vi "Addon.Dialog.vi"(8 "error in (no error)":errorcluster) -> (0 "error out":errorcluster, 2 "Diagnostics Basic Configuration":T1, 3 "Cancelled?":bool)   [LabVIEW 2024, in "Diagnostics Addon System Explorer.lvlib"]
uses:
  Diagnostics Addon System Explorer.lvlib
  Addon Shared/Types/Protocol.ctl
  Types/Addon.Initialize.ctl
  Addon Shared/Diagnostics Addon Shared.lvlib
panel:
  in  "Baud Rate":u32=250000
  in  "Path":path caption="Previous Personality Path (Optional)"
  in  "Cancel":bool
  in  "OK":bool
  in  "Diagnostic Protocol":T2
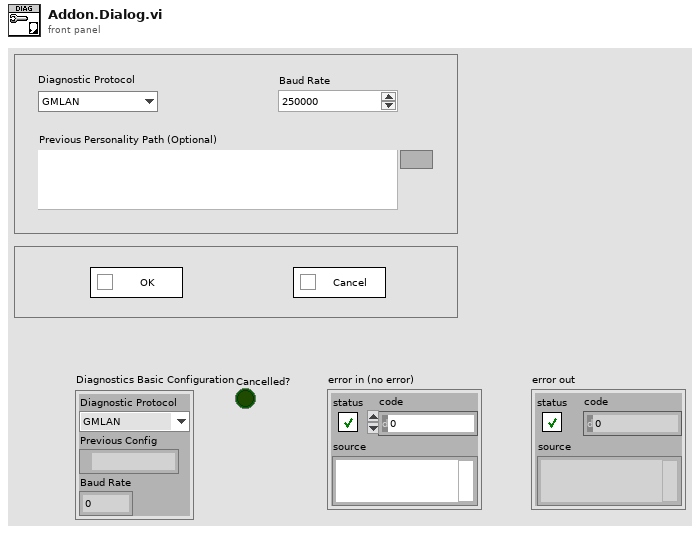
[diagram p1: front panel]
types:
  T1 = typedef "Diagnostics Addon System Explorer.lvlib/Addon.Initialize.ctl" = cluster{"Diagnostic Protocol":T2, "Previous Config":path, "Baud Rate":u32}
  T2 = typedef "Diagnostics Addon Shared.lvlib/Protocol.ctl" = enum16{"GMLAN", "KWP-2000", "UDS", "User-Defined"}
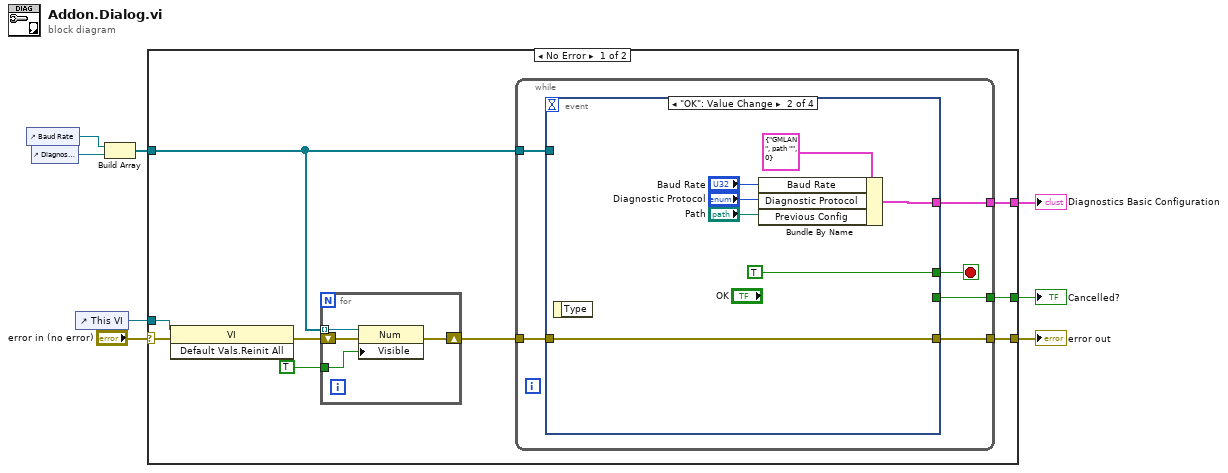
[diagram p0: block diagram]
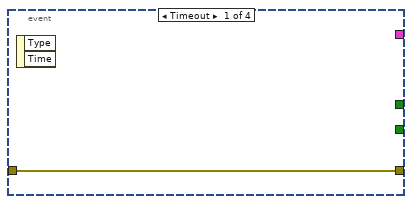
[diagram p2: hidden frame]
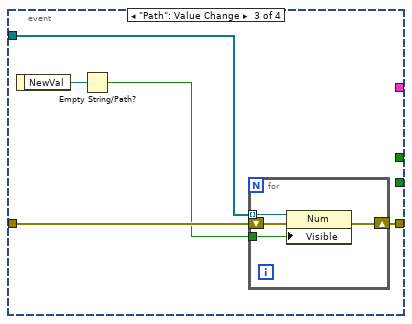
[diagram p3: hidden frame]
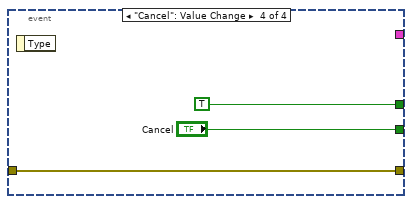
[diagram p4: hidden frame]
diagram:
  n1 = control-ref of="Baud Rate"() -> (w1:refnum<vi>)
  n2 = control-ref of="Diagnostic Protocol"() -> (w3:refnum<vi>)
  n3 = control-ref of="This VI"() -> (w4:refnum<vi>)
  n4 = Build Array(w1, w3) -> (w2:refnum<vi>[])
  n5 = case shown="No Error" "error in (no error)" {
    selector: "error in (no error)" -> [w14 w48]
    tunnel: [w17 _] -> w8
    tunnel: [w16 _] -> w7
    tunnel: [w13 w48] -> w5
    tunnel: w4 -> [w15 _]
    tunnel: w2 -> [w10 _]
    frame No Error {
      n6 = invoke class="VI" method="Default Vals.Reinit All"(reference=w15, error in=w14) -> (error out=w12:errorcluster)  [unwired: 1 in, 2 out]
      n7 = for {
        tunnel: w10 -> [w21] mode=indexing
        shift-right: [w19] -> w11
        shift-left: w12 -> [w20]
        tunnel: TRUE -> [w18]
        n8 = property class="Num"(reference=w21, error in=w20, "Visible"=w18) -> (error out=w19:errorcluster)  [unwired: 1 out]
      }
      n9 = while {
        tunnel: [w27] -> w17
        tunnel: [w25] -> w16
        tunnel: [w23] -> w13
        tunnel: w11 -> [w24]
        tunnel: w10 -> [w22]
        stop <- w26 stop-if-true
        n10 = event shown="[1] \"OK\": Value Change" {
          selector: _ -> [_ _ _ _]
          dyn-events: _ -> [_ _ _ _]
          timeout: _ -> [_ _ _ _]
          tunnel: [_ _ _ "Cancel"] -> w27
          tunnel: [_ TRUE _ TRUE] -> w26
          tunnel: [_ w33 _ _] -> w25
          tunnel: w24 -> [w28 w31 w39 w45]
          tunnel: [w28 w31 w38 w45] -> w23
          tunnel: w22 -> [_ _ w37 _]
          event Timeout {
            n11 = event-data() -> ()  [unwired: 1 in, 2 out]
          }
          event "OK": Value Change {
            n12 = event-data() -> ()  [unwired: 1 in, 1 out]
            n13 = Bundle By Name(cluster=T1 {"Diagnostic Protocol"=enum."GMLAN", "Previous Config"=path "", "Baud Rate"=0} ("output cluster"), "Baud Rate"="Baud Rate", "Diagnostic Protocol"="Diagnostic Protocol", "Previous Config"="Path") -> (w33:T1)
          }
          event "Path": Value Change {
            n14 = event-data() -> ("NewVal"=w40:path)  [unwired: 1 in]
            n15 = Empty String/Path?(string/path=w40) -> (empty?=w36:bool)
            n16 = for {
              tunnel: w37 -> [w44] mode=indexing
              shift-right: [w42] -> w38
              shift-left: w39 -> [w43]
              tunnel: w36 -> [w41]
              n17 = property class="Num"(reference=w44, error in=w43, "Visible"=w41) -> (error out=w42:errorcluster)  [unwired: 1 out]
            }
          }
          event "Cancel": Value Change {
            n18 = event-data() -> ()  [unwired: 1 in, 1 out]
          }
        }
      }
    }
    frame Error {
    }
  }
  "Cancelled?" <- w8
  "Diagnostics Basic Configuration" <- w7
  "error out" <- w5
